vi "Client.vi"() -> ()   [LabVIEW 2015]
uses:
  <vilib>/Platform/TimedLoop/XDataNode/timing_clust.ctl
  <vilib>/Platform/TimedLoop/XDataNode/nitl_modes.ctl
  <vilib>/Platform/TimedLoop/XDataNode/wakeup.ctl
  <vilib>/platform/TimedLoop/XDataNode/XDataNode.xnode
  <vilib>/Platform/TimedLoop/XDataNode/XDNodeRunTimeDep.lvlib
panel:
  out "output cluster":T1
  out "Time":u32
  out "Counter":i32
  # "Overview:  Coding that exemplifies how to benchmark the communication of Shared Variables.\nRequirements: LabVIEW 2012 or compatible\nInstructions:\n1. Run this VI\n2. Watch the amount of time it takes to communicate on the \"Benchmark SV Send  LV2012 - NI Verified.vi\" \n3. Stop both VIs"
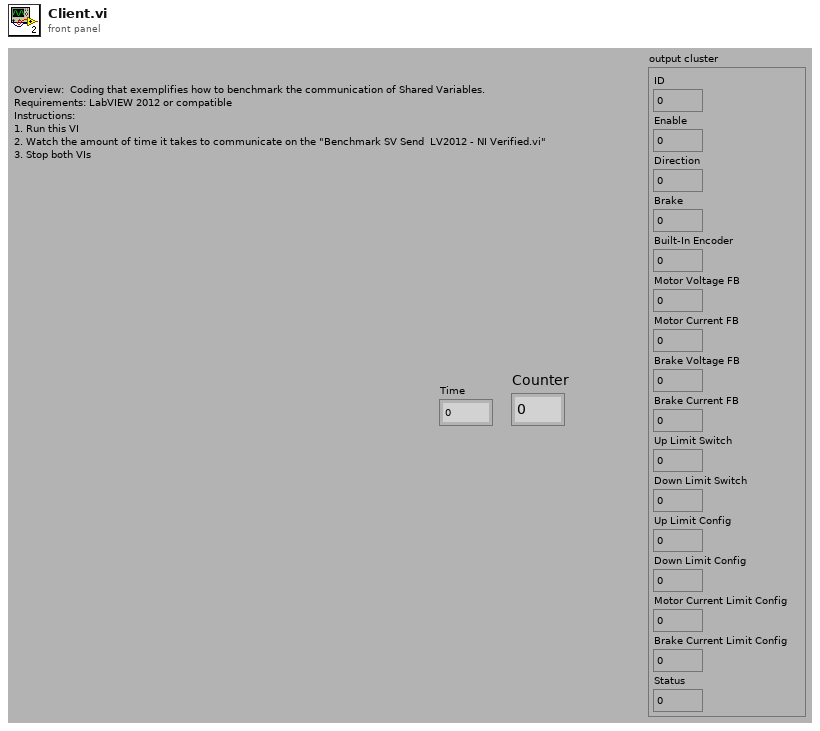
[diagram p1: front panel]
types:
  T1 = cluster{"ID":dbl, "Enable":dbl, "Direction":dbl, "Brake":dbl, "Built-In Encoder":dbl, "Motor Voltage FB":dbl, "Motor Current FB":dbl, "Brake Voltage FB":dbl, "Brake Current FB":dbl, "Up Limit Switch":dbl, "Down Limit Switch":dbl, "Up Limit Config":dbl, "Down Limit Config":dbl, "Motor Current Limit Config":dbl, "Brake Current Limit Config":dbl, "Status":dbl}
  T2 = typedef "XDNodeRunTimeDep.lvlib/timing_clust.ctl" = cluster{"Expected End [f-1]":u64, "Actual End [f-1]":u64, "Finished Late? [f-1]":bool, "Expected End [i-1]":u64, "Actual End [i-1]":u64, "Finished Late? [i-1]":bool, "Expected Start [i]":u64, "Actual Start [i]":u64, "Expected Start [f]":u64, "Actual Start [f]":u64, "Source Name":string, "Structure Name":string, "Period":i64, "Deadline":i64, "Offset":i64, "Start":i64, "Priority":i32, "Timeout":i32, "Mode":T3, "Wakeup Reason":T4, "Error":errorcluster, "Source Type":string, "Secondary Source Type":string, "Global End Time":u64, "Global Start Time":u64, "Frame Duration":u64, "Iteration Duration":u64, "Assigned CPU":i32, "I/O Scan Engine Mode":u32}
  T3 = typedef "XDNodeRunTimeDep.lvlib/nitl_modes.ctl" = enum32{"No Change", "Process missed periods, maintain original phase", "Discard missed periods, maintain original phase", "Process missed periods, ignore original phase", "Discard missed periods, ignore original phase"}
  T4 = typedef "XDNodeRunTimeDep.lvlib/wakeup.ctl" = enum32{"Normal", "Aborted", "Asynchronous wakeup", "Timing source error", "Timed loop error", "Timeout"}
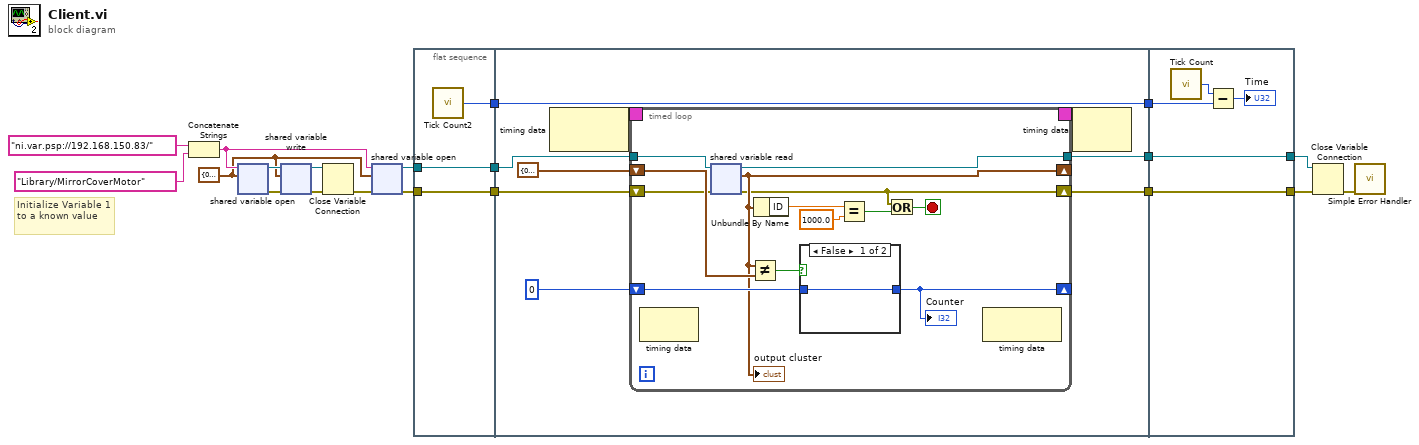
[diagram p0: block diagram]
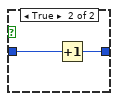
[diagram p2: hidden frame]
diagram:
  w2 = T1 {"ID"=0.0, "Enable"=0.0, "Direction"=0.0, "Brake"=0.0, "Built-In Encoder"=0.0, "Motor Voltage FB"=0.0, "Motor Current FB"=0.0, "Brake Voltage FB"=0.0, "Brake Current FB"=0.0, "Up Limit Switch"=0.0, "Down Limit Switch"=0.0, "Up Limit Config"=0.0, "Down Limit Config"=0.0, "Motor Current Limit Config"=0.0, "Brake Current Limit Config"=0.0, "Status"=0.0} ("MirrorCoverMotor")
  # "Initialize Variable 1 to a known value"
  n1 = Concatenate Strings("ni.var.psp://192.168.150.83/" ("string"), "Library/MirrorCoverMotor") -> (w6:string)
  n2 = shared-variable-open(w6, w2) -> (w5:refnum<k21>, w8:errorcluster)  [unwired: 2 in]
  n3 = shared-variable-write(w5, w8, w2) -> (w4:refnum<k21>, w7:errorcluster)
  n4 = Close Variable Connection(8:w7, 11:w4) -> (0:w3:errorcluster)
  n5 = shared-variable-open(w6, w3, w2) -> (w17:refnum<k21>, w18:errorcluster)  [unwired: 1 in]
  n6 = flat-sequence {
    tunnel: w17 -> [w22]
    tunnel: w18 -> [w23]
    tunnel: [w23] -> w11
    tunnel: [w22] -> w10
    tunnel: [w21] -> w9
    tunnel: [w29] -> w16
    tunnel: [w28] -> w15
    tunnel: [w24] -> w14
    tunnel: w11 -> [w32]
    tunnel: w10 -> [w31]
    tunnel: w9 -> [w24]
    tunnel: w16 -> [w53]
    tunnel: w15 -> [w54]
    tunnel: w14 -> [w55]
    tunnel: [w54] -> w13
    tunnel: [w53] -> w12
    frame #0 {
      n7 = call "Tick Count2"() -> ("Tick Count(mSec)"=w21:u32)
    }
    frame #1 {
      n8 = node-c288() -> (w27:T2)  [unwired: 1 in]
      n9 = timed-loop {
        shift-right: [w38] -> _
        shift-left: T1 {"ID"=0.0, "Enable"=0.0, "Direction"=0.0, "Brake"=0.0, "Built-In Encoder"=0.0, "Motor Voltage FB"=0.0, "Motor Current FB"=0.0, "Brake Voltage FB"=0.0, "Brake Current FB"=0.0, "Up Limit Switch"=0.0, "Down Limit Switch"=0.0, "Up Limit Config"=0.0, "Down Limit Config"=0.0, "Motor Current Limit Config"=0.0, "Brake Current Limit Config"=0.0, "Status"=0.0} ("MirrorCoverMotor") -> [w45]
        shift-right: [w35] -> w29
        shift-left: w32 -> [w42]
        shift-right: [w39] -> _
        shift-left: 0 -> [w44]
        tunnel: w31 -> [w43]
        tunnel: [w41] -> w28
        timing: w27 -> [_]
        timing-out: [_] -> w26
        stop <- w33 stop-if-true
        n10 = node-c288() -> ()  [unwired: 1 in, 1 out]
        n11 = shared-variable-read(w43, w42) -> (w41:refnum<k21>, w35:errorcluster, w38:T1)  [unwired: 1 out]
        "output cluster" <- w38
        n12 = Not Equal?(x=w38, y=w45) -> (x != y?=w40:bool)
        n13 = Unbundle By Name(w38) -> ("ID"=w37:dbl)
        n14 = case shown="False" w40 {
          tunnel: w44 -> [w48 w50]
          tunnel: [w48 w49] -> w39
          frame False {
          }
          frame True {
            n15 = Increment(x=w50) -> (x+1=w49:i32)
          }
        }
        "Counter" <- w39
        n16 = Equal?(x=w37, y=1000.0) -> (x = y?=w34:bool)
        n17 = Or(x=w35, y=w34) -> (x .or. y?=w33:bool)
        n18 = node-c288() -> ()  [unwired: 1 in, 1 out]
      }
      n19 = node-c288(w26) -> ()  [unwired: 1 out]
    }
    frame #2 {
      n20 = call "Tick Count"() -> ("Tick Count(mSec)"=w57:u32)
      n21 = Subtract(x=w57, y=w55) -> (x-y=→"Time":u32)
    }
  }
  n22 = Close Variable Connection(8:w12, 11:w13) -> (0:w1:errorcluster)
  n23 = call <vilib>:"Simple Error Handler.vi"("error in (no error)"=w1) -> ()  [unwired: 4 in, 5 out]
